vi "munormalizada.vi"(4 "Array":u32[][](array[numeric])) -> (14 "un02":dbl, 18 "un03":dbl, 19 "un30":dbl, 21 "un11":dbl, 23 "un12":dbl, 25 "un20":dbl, 27 "un21":dbl)   [LabVIEW 2021]
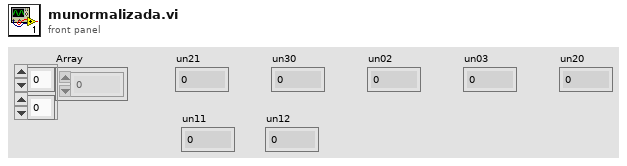
[diagram p1: front panel]
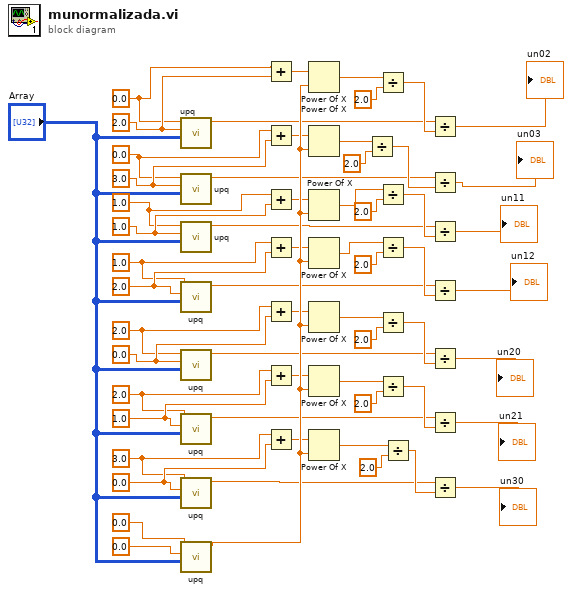
[diagram p0: block diagram]
diagram:
  w19 = 2.0 ("q")
  w18 = 0.0 ("p")
  w28 = 3.0 ("q")
  w27 = 0.0 ("p")
  w30 = 1.0 ("q")
  w29 = 1.0 ("p")
  w38 = 0.0 ("q")
  w37 = 3.0 ("p")
  w36 = 1.0 ("q")
  w35 = 2.0 ("p")
  w34 = 0.0 ("q")
  w33 = 2.0 ("p")
  w32 = 2.0 ("q")
  w31 = 1.0 ("p")
  n1 = call "upq.vi"("ImagenBinaria"="Array", "q"=w19, "p"=w18) -> ("upq"=w4:dbl)  [unwired: 8 in]
  n2 = call "upq.vi"("ImagenBinaria"="Array", "q"=w28, "p"=w27) -> ("upq"=w5:dbl)  [unwired: 8 in]
  n3 = call "upq.vi"("ImagenBinaria"="Array", "q"=w30, "p"=w29) -> ("upq"=w9:dbl)  [unwired: 8 in]
  n4 = call "upq.vi"("ImagenBinaria"="Array", "q"=w32, "p"=w31) -> ("upq"=w3:dbl)  [unwired: 8 in]
  n5 = call "upq.vi"("ImagenBinaria"="Array", "q"=w34, "p"=w33) -> ("upq"=w6:dbl)  [unwired: 8 in]
  n6 = call "upq.vi"("ImagenBinaria"="Array", "q"=w36, "p"=w35) -> ("upq"=w7:dbl)  [unwired: 8 in]
  n7 = call "upq.vi"("ImagenBinaria"="Array", "q"=w38, "p"=w37) -> ("upq"=w8:dbl)  [unwired: 8 in]
  n8 = call "upq.vi"("ImagenBinaria"="Array", "q"=0.0, "p"=0.0) -> ("upq"=w39:dbl)  [unwired: 8 in]
  n9 = Add(x=w18, y=w19) -> (x+y=w20:dbl)
  n10 = Add(x=w27, y=w28) -> (x+y=w21:dbl)
  n11 = Add(x=w29, y=w30) -> (x+y=w22:dbl)
  n12 = Add(x=w31, y=w32) -> (x+y=w23:dbl)
  n13 = Add(x=w33, y=w34) -> (x+y=w24:dbl)
  n14 = Add(x=w35, y=w36) -> (x+y=w25:dbl)
  n15 = Add(x=w37, y=w38) -> (x+y=w26:dbl)
  n16 = Power Of X(1:w39, 2:w20) -> (0:w43:dbl)
  n17 = Power Of X(1:w39, 2:w21) -> (0:w45:dbl)
  n18 = Power Of X(1:w39, 2:w22) -> (0:w47:dbl)
  n19 = Power Of X(1:w39, 2:w23) -> (0:w53:dbl)
  n20 = Power Of X(1:w39, 2:w24) -> (0:w55:dbl)
  n21 = Power Of X(1:w39, 2:w25) -> (0:w57:dbl)
  n22 = Power Of X(1:w39, 2:w26) -> (0:w59:dbl)
  n23 = Divide(x=w45, y=2.0) -> (x/y=w46:dbl)
  n24 = Divide(x=w43, y=2.0) -> (x/y=w44:dbl)
  n25 = Divide(x=w47, y=2.0) -> (x/y=w48:dbl)
  n26 = Divide(x=w53, y=2.0) -> (x/y=w54:dbl)
  n27 = Divide(x=w55, y=2.0) -> (x/y=w56:dbl)
  n28 = Divide(x=w57, y=2.0) -> (x/y=w58:dbl)
  n29 = Divide(x=w59, y=2.0) -> (x/y=w60:dbl)
  n30 = Divide(x=w4, y=w44) -> (x/y=→"un02":dbl)
  n31 = Divide(x=w5, y=w46) -> (x/y=→"un03":dbl)
  n32 = Divide(x=w9, y=w48) -> (x/y=→"un11":dbl)
  n33 = Divide(x=w3, y=w54) -> (x/y=→"un12":dbl)
  n34 = Divide(x=w6, y=w56) -> (x/y=→"un20":dbl)
  n35 = Divide(x=w7, y=w58) -> (x/y=→"un21":dbl)
  n36 = Divide(x=w8, y=w60) -> (x/y=→"un30":dbl)
